vi "DAQ Configuration.vi"(8 "error in (no error)":errorcluster, 10 "DAQ Configuration":T1(ring), 11 "Settings in":refnum<class "Settings.lvclass">) -> (0 "error out":errorcluster, 3 "Settings out":refnum<class "Settings.lvclass">)   [LabVIEW 2023, in "GUI.lvlib" / "Settings.lvlib" / "Settings.lvclass"]
uses:
  Settings.lvclass
  Settings.lvclass/Settings.ctl
  HardwareAbstractionLayer_LVOOP/Database/Database.lvclass
panel:
  out "PhysicalChannel":string
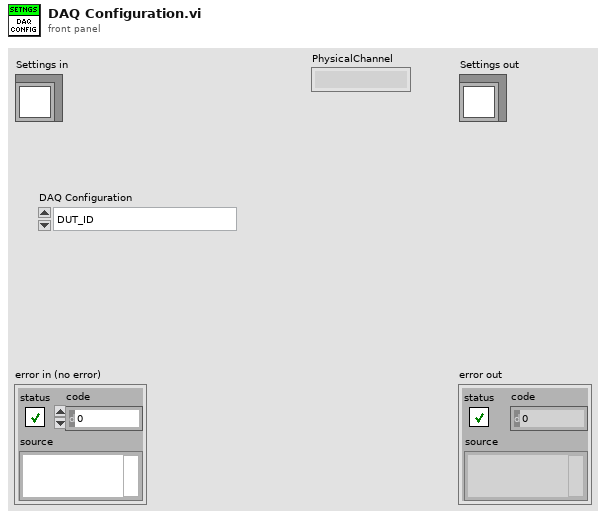
[diagram p1: front panel]
types:
  T1 = enum16{"DUT_ID", "Channel Type", "Search", "Update", "Double Click"}
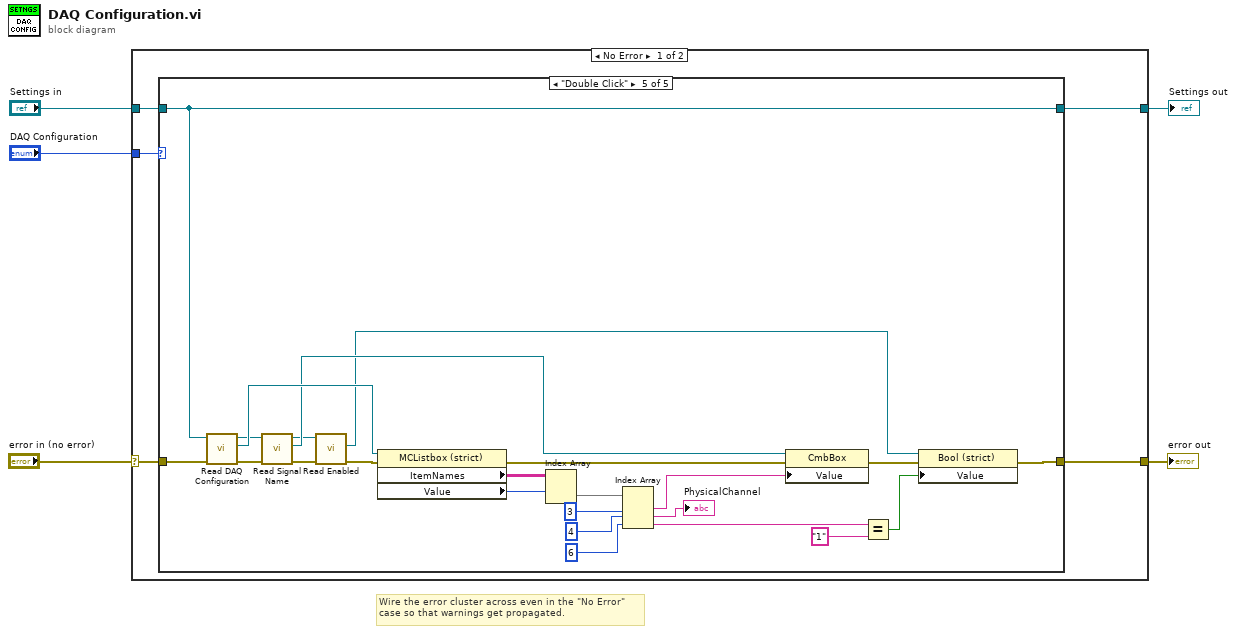
[diagram p0: block diagram]
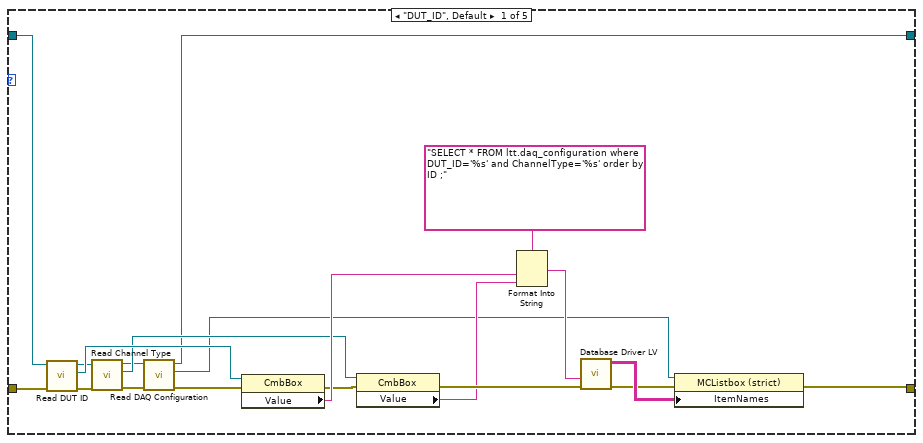
[diagram p2: hidden frame]
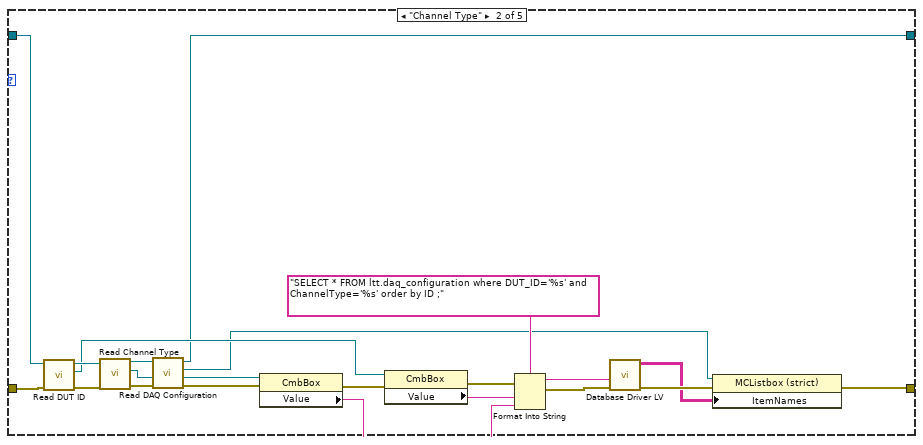
[diagram p3: hidden frame]
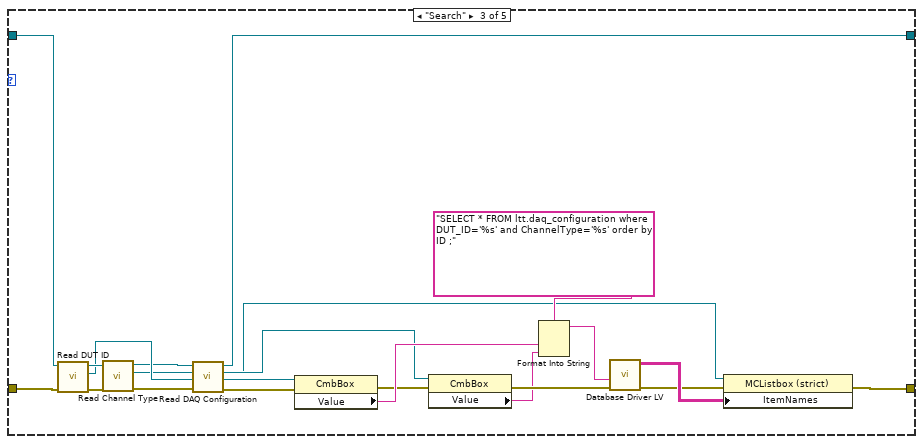
[diagram p4: hidden frame]
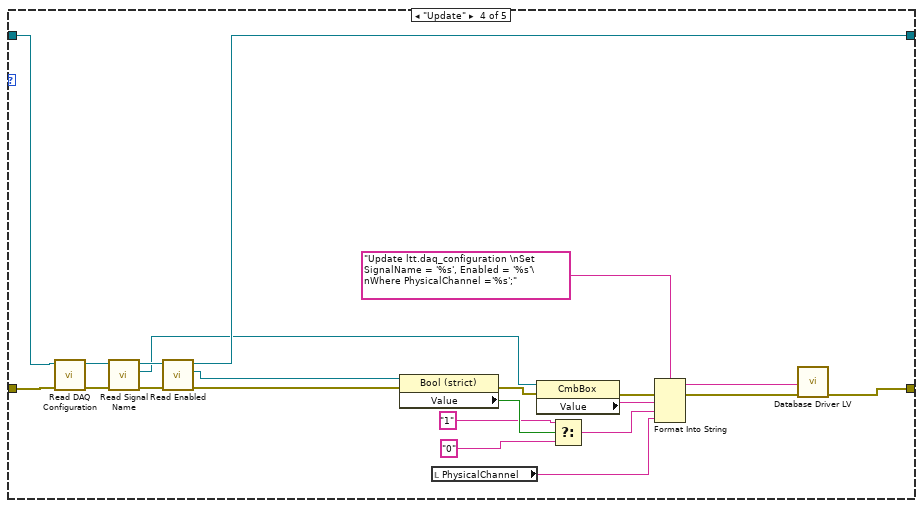
[diagram p5: hidden frame]
diagram:
  # "Wire the error cluster across even in the \"No Error\"\ncase so that warnings get propagated."
  n1 = case shown="No Error" "error in (no error)" {
    selector: "error in (no error)" -> [w10 w119]
    tunnel: [w6 w119] -> w4
    tunnel: [w7 w118] -> w2
    tunnel: "Settings in" -> [w8 w118]
    tunnel: "DAQ Configuration" -> [w9 _]
    frame No Error {
      n2 = case shown="\"Double Click\"" w9 {
        tunnel: w10 -> [w18 w44 w64 w82 w105]
        tunnel: [w12 w31 w53 w76 w104] -> w7
        tunnel: w8 -> [w24 w42 w61 w83 w104]
        tunnel: [w16 w40 w62 w72 w95] -> w6
        frame "DUT_ID", Default {
          n3 = call "Read DUT ID.vi"("error in (no error)"=w18, "Settings in"=w24) -> ("error out"=w21:errorcluster, "DUT ID"=w23:refnum<vi>, "Settings out"=w20:refnum<class "Settings.lvclass">)  [unwired: 7 in]
          n4 = call "Read Channel Type.vi"("error in (no error)"=w21, "Settings in"=w20) -> ("error out"=w14:errorcluster, "Channel Type"=w19:refnum<vi>, "Settings out"=w15:refnum<class "Settings.lvclass">)  [unwired: 7 in]
          n5 = call "Read DAQ Configuration .vi"("error in (no error)"=w14, "Settings in"=w15) -> ("error out"=w13:errorcluster, "DAQ Configuration"=w11:refnum<vi>, "Settings out"=w12:refnum<class "Settings.lvclass">)  [unwired: 7 in]
          n6 = property on="Property Node" class="CmbBox"(reference=w23, error in=w13) -> (error out=w17:errorcluster, "Value"=w22:string)  [unwired: 1 out]
          n7 = property on="Property Node" class="CmbBox"(reference=w19, error in=w17) -> (error out=w26:errorcluster, "Value"=w25:string)  [unwired: 1 out]
          n8 = Format Into String(format string="SELECT * FROM ltt.daq_configuration where DUT_ID='%s' and ChannelType='%s' order by ID ;", w22, w25) -> (resulting string=w29:string)  [unwired: 2 in, 1 out]
          n9 = call "Database Driver LV.vi"("error in"=w26, "SQL query"=w29) -> ("error out"=w27:errorcluster, "data"=w28:string[][])  [unwired: 6 in, 2 out]
          n10 = property on="Property Node" class="MCListbox (strict)"(reference=w11, error in=w27, "ItemNames"=w28) -> (error out=w16:errorcluster)  [unwired: 1 out]
        }
        frame "Channel Type" {
          n11 = call "Read DUT ID.vi"("error in (no error)"=w44, "Settings in"=w42) -> ("error out"=w43:errorcluster, "DUT ID"=w38:refnum<vi>, "Settings out"=w41:refnum<class "Settings.lvclass">)  [unwired: 7 in]
          n12 = call "Read Channel Type.vi"("error in (no error)"=w43, "Settings in"=w41) -> ("error out"=w34:errorcluster, "Channel Type"=w37:refnum<vi>, "Settings out"=w35:refnum<class "Settings.lvclass">)  [unwired: 7 in]
          n13 = call "Read DAQ Configuration .vi"("error in (no error)"=w34, "Settings in"=w35) -> ("error out"=w33:errorcluster, "DAQ Configuration"=w32:refnum<vi>, "Settings out"=w31:refnum<class "Settings.lvclass">)  [unwired: 7 in]
          n14 = property on="Property Node" class="CmbBox"(reference=w37, error in=w33) -> (error out=w39:errorcluster, "Value"=w36:string)  [unwired: 1 out]
          n15 = property on="Property Node" class="CmbBox"(reference=w38, error in=w39) -> (error out=w47:errorcluster, "Value"=w45:string)  [unwired: 1 out]
          n16 = Format Into String(format string="SELECT * FROM ltt.daq_configuration where DUT_ID='%s' and ChannelType='%s' order by ID ;", error in=w47, w45, w36) -> (resulting string=w48:string, error out=w46:errorcluster)  [unwired: 1 in]
          n17 = call "Database Driver LV.vi"("error in"=w46, "SQL query"=w48) -> ("error out"=w51:errorcluster, "data"=w50:string[][])  [unwired: 6 in, 2 out]
          n18 = property on="Property Node" class="MCListbox (strict)"(reference=w32, error in=w51, "ItemNames"=w50) -> (error out=w40:errorcluster)  [unwired: 1 out]
        }
        frame "Search" {
          n19 = call "Read DUT ID.vi"("error in (no error)"=w64, "Settings in"=w61) -> ("error out"=w63:errorcluster, "DUT ID"=w58:refnum<vi>, "Settings out"=w60:refnum<class "Settings.lvclass">)  [unwired: 7 in]
          n20 = call "Read Channel Type.vi"("error in (no error)"=w63, "Settings in"=w60) -> ("error out"=w55:errorcluster, "Channel Type"=w57:refnum<vi>, "Settings out"=w56:refnum<class "Settings.lvclass">)  [unwired: 7 in]
          n21 = call "Read DAQ Configuration .vi"("error in (no error)"=w55, "Settings in"=w56) -> ("error out"=w54:errorcluster, "DAQ Configuration"=w52:refnum<vi>, "Settings out"=w53:refnum<class "Settings.lvclass">)  [unwired: 7 in]
          n22 = property on="Property Node" class="CmbBox"(reference=w58, error in=w54) -> (error out=w59:errorcluster, "Value"=w71:string)  [unwired: 1 out]
          n23 = property on="Property Node" class="CmbBox"(reference=w57, error in=w59) -> (error out=w67:errorcluster, "Value"=w66:string)  [unwired: 1 out]
          n24 = Format Into String(format string="SELECT * FROM ltt.daq_configuration where DUT_ID='%s' and ChannelType='%s' order by ID ;", w71, w66) -> (resulting string=w70:string)  [unwired: 2 in, 1 out]
          n25 = call "Database Driver LV.vi"("error in"=w67, "SQL query"=w70) -> ("error out"=w68:errorcluster, "data"=w69:string[][])  [unwired: 6 in, 2 out]
          n26 = property on="Property Node" class="MCListbox (strict)"(reference=w52, error in=w68, "ItemNames"=w69) -> (error out=w62:errorcluster)  [unwired: 1 out]
        }
        frame "Update" {
          n27 = call "Read DAQ Configuration .vi"("error in (no error)"=w82, "Settings in"=w83) -> ("error out"=w79:errorcluster, "Settings out"=w78:refnum<class "Settings.lvclass">)  [unwired: 7 in, 1 out]
          n28 = call "Read Signal Name.vi"("error in (no error)"=w79, "Settings in"=w78) -> ("error out"=w80:errorcluster, "Signal Name"=w74:refnum<vi>, "Settings out"=w77:refnum<class "Settings.lvclass">)  [unwired: 7 in]
          n29 = call "Read Enabled.vi"("error in (no error)"=w80, "Settings in"=w77) -> ("error out"=w73:errorcluster, "Enabled"=w75:refnum<vi>, "Settings out"=w76:refnum<class "Settings.lvclass">)  [unwired: 7 in]
          n30 = property on="Property Node" class="Bool (strict)"(reference=w75, error in=w73) -> (error out=w89:errorcluster, "Value"=w88:bool)  [unwired: 1 out]
          n31 = local read "PhysicalChannel"() -> (w81:string)
          n32 = property on="Property Node" class="CmbBox"(reference=w74, error in=w89) -> (error out=w90:errorcluster, "Value"=w92:string)  [unwired: 1 out]
          n33 = Select(t="1", s=w88, f="0") -> (s? t:f=w86:string)
          n34 = Format Into String(format string="Update ltt.daq_configuration \nSet SignalName = '%s', Enabled = '%s'\nWhere PhysicalChannel ='%s';", error in=w90, w92, w86, w81) -> (resulting string=w84:string, error out=w91:errorcluster)  [unwired: 1 in]
          n35 = call "Database Driver LV.vi"("error in"=w91, "SQL query"=w84) -> ("error out"=w72:errorcluster)  [unwired: 6 in, 3 out]
        }
        frame "Double Click" {
          n36 = call "Read DAQ Configuration .vi"("error in (no error)"=w105, "Settings in"=w104) -> ("error out"=w102:errorcluster, "DAQ Configuration"=w103:refnum<vi>, "Settings out"=w101:refnum<class "Settings.lvclass">)  [unwired: 7 in]
          n37 = call "Read Signal Name.vi"("error in (no error)"=w102, "Settings in"=w101) -> ("error out"=w99:errorcluster, "Signal Name"=w100:refnum<vi>, "Settings out"=w98:refnum<class "Settings.lvclass">)  [unwired: 7 in]
          n38 = call "Read Enabled.vi"("error in (no error)"=w99, "Settings in"=w98) -> ("error out"=w96:errorcluster, "Enabled"=w97:refnum<vi>)  [unwired: 7 in, 1 out]
          n39 = property on="Property Node" class="MCListbox (strict)"(reference=w103, error in=w96) -> (error out=w113:errorcluster, "ItemNames"=w117:string[][], "Value"=w94:i32)  [unwired: 1 out]
          n40 = Index Array(array=w117, index (row)=w94) -> (element=w116:string[])  [unwired: 1 in]
          n41 = Index Array(array=w116, index #1=3 ("index"), index #2=4 ("index"), index #3=6 ("index")) -> (element #1=w114:string, element #2=→"PhysicalChannel":string, element #3=w107:string)
          n42 = property on="Property Node" class="CmbBox"(reference=w100, error in=w113, "Value"=w114) -> (error out=w111:errorcluster)  [unwired: 1 out]
          n43 = Equal?(x=w107, y="1") -> (x = y?=w110:bool)
          n44 = property on="Property Node" class="Bool (strict)"(reference=w97, error in=w111, "Value"=w110) -> (error out=w95:errorcluster)  [unwired: 1 out]
        }
      }
    }
    frame Error {
    }
  }
  "error out" <- w4
  "Settings out" <- w2
